vi "室外视频预览.vi"() -> ()   [LabVIEW 2018]
doc: "This example shows how to open, read, and display an AVI file in NI Vision. The VI reads the frames per second property and plays the images back at the rate specified by the AVI file."
uses:
  <vilib>/Utility/error.llb/DialogType.ctl
panel:
  out "数值输入控件":i32
  in  "重新读取":bool
  out "视频的帧数：":u32
  out "Path":path
  out "添加的路径":path
  out "视频预览":T1(plugin-control)
  in  "Stop 2":bool
  out "Progress Bar 2":i32(slide) max=41 scale=-1.0..41.0
  in  "下一步":bool
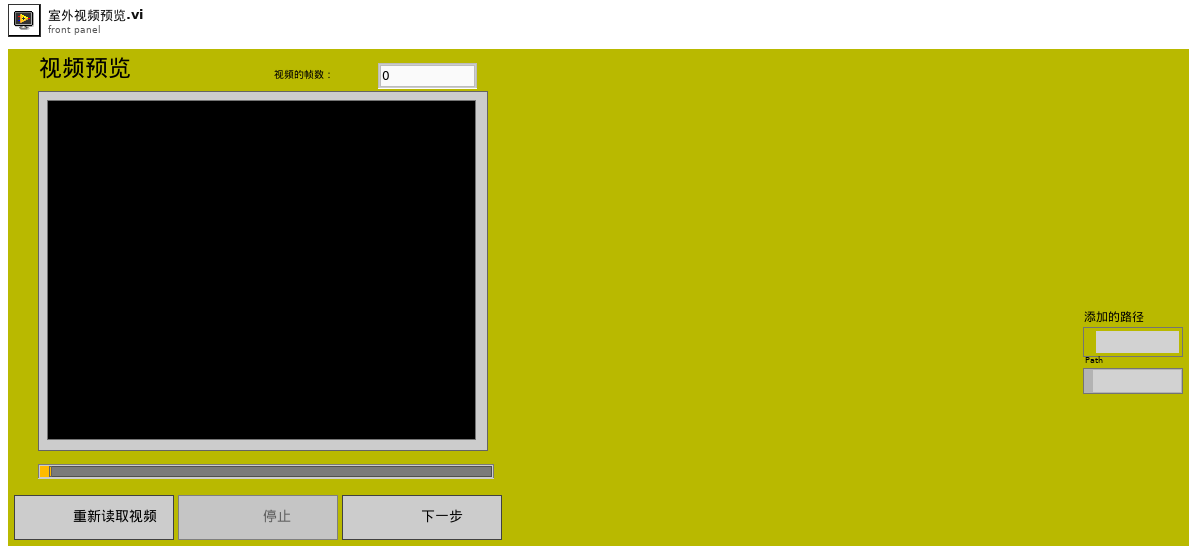
[diagram p1: front panel]
types:
  T1 = typedef "IMAQ Image.ctl" = refnum<image>
  T2 = enum8{"Enabled", "Disabled", "Disabled and Grayed Out"}
  T3 = enum32{"Invalid", "Standard", "Closed", "Hidden", "Minimized", "Maximized"}
  T4 = typedef "DialogType.ctl" = u16
  T5 = typedef "IMAQ AVI2 Refnum.ctl" = refnum<k20>
  T6 = typedef "Image Type" = u32
  T7 = cluster{"Width":u32, "Height":u32, "Frames Per Second":u32, "Codec":string, "Has Data":bool}
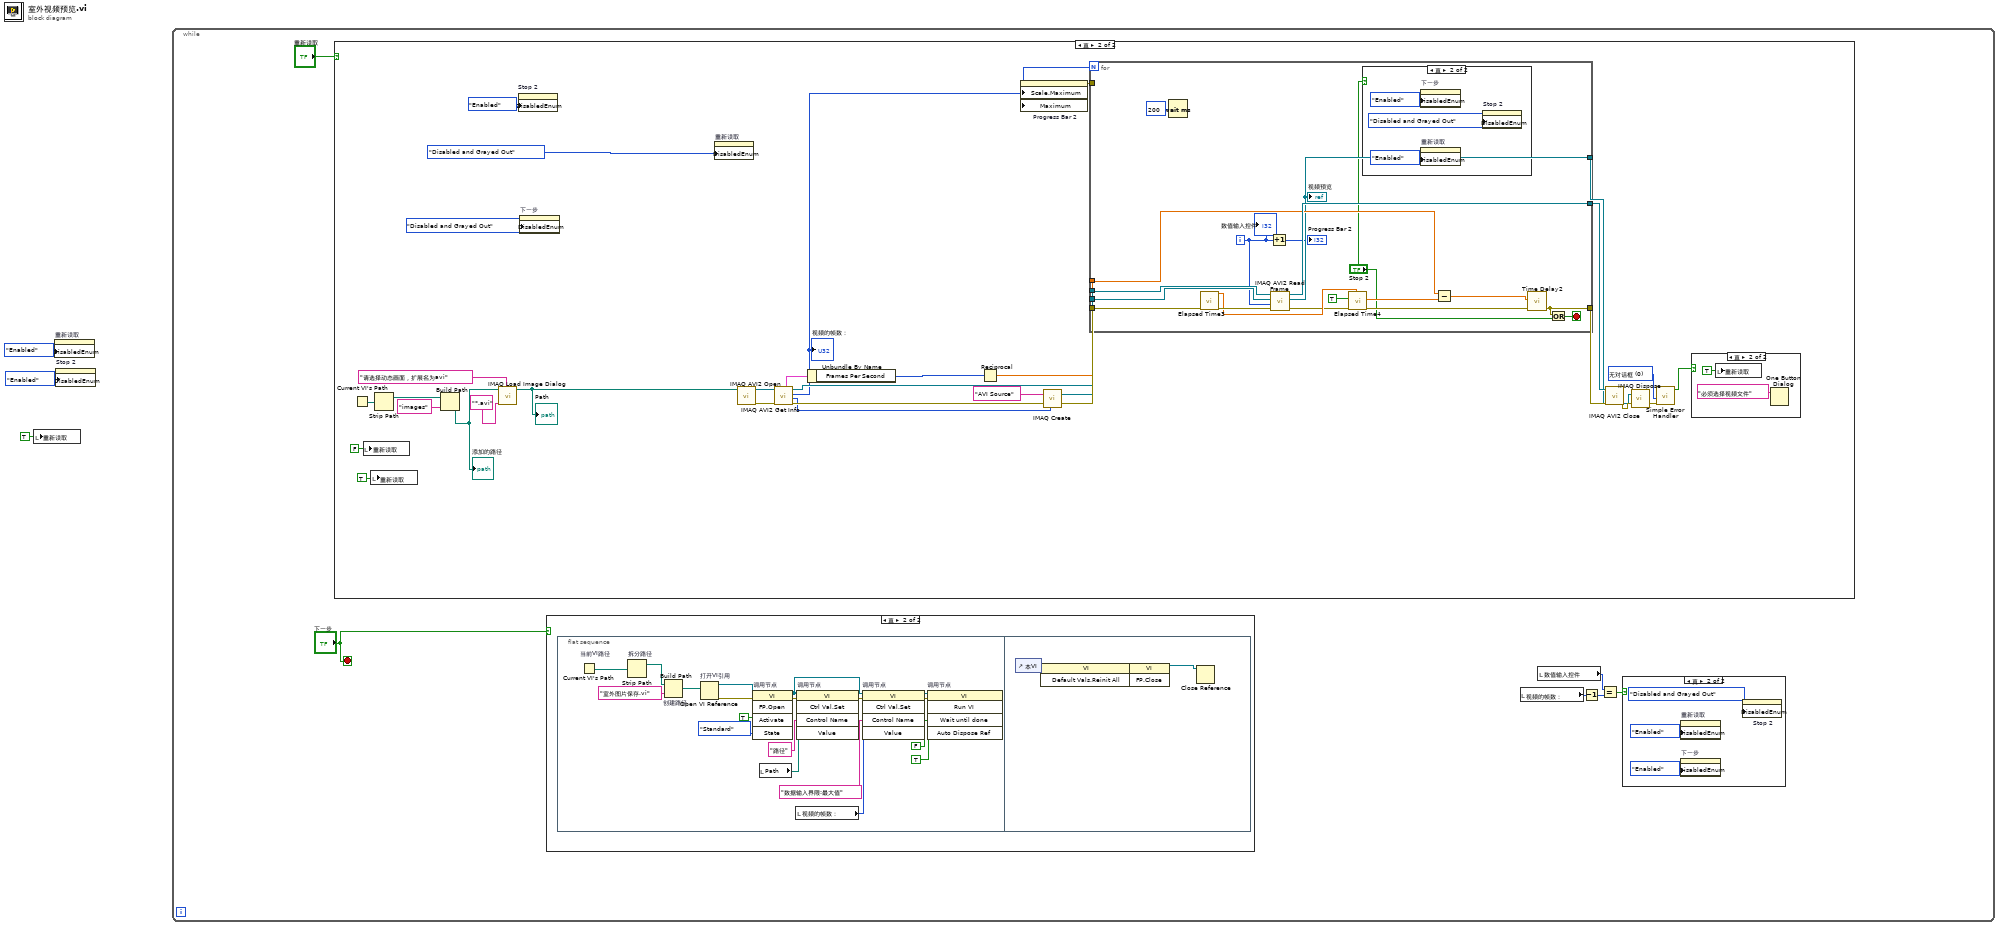
[diagram p0: block diagram]
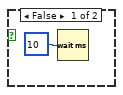
[diagram p6: hidden frame]
diagram:
  n1 = local write "重新读取"(TRUE ("布尔")) -> ()
  n2 = property on="重新读取" class="Bool (严格)"("DisabledEnum"=T2."Enabled" ("禁用")) -> ()  [unwired: 2 in, 2 out]
  n3 = property on="Stop 2" class="Bool"("DisabledEnum"=T2."Enabled" ("禁用")) -> ()  [unwired: 2 in, 2 out]
  n4 = while {
    stop <- "下一步" stop-if-true
    n5 = case shown="真" "重新读取" {
      frame False {
      }
      frame True {
        w19 = T4 0 items=["无对话框", "确定信息", "继续或停止信息", "确定信息＋警告", "继续/停止+警告"] ("type of dialog (OK msg:1)")
        n6 = Current VI's Path() -> (path=w23:path)
        n7 = local write "重新读取"(FALSE ("布尔")) -> ()
        n8 = local write "重新读取"(TRUE ("布尔")) -> ()
        n9 = Strip Path(path=w23) -> (stripped path=w22:path)  [unwired: 1 out]
        n10 = Build Path(base path=w22, name or relative path="images") -> (appended path=w26:path)
        "添加的路径" <- w26
        n11 = call "IMAQ Load Image Dialog"("Prompt"="请选择动态画面，扩展名为avi" ("prompt"), "Pattern"="*.avi", "Start Path"=w26) -> ("Path"=w20:path)  [unwired: 6 in, 2 out]
        "Path" <- w20
        n12 = property on="Stop 2" class="Bool"("DisabledEnum"=T2."Enabled" ("禁用")) -> ()  [unwired: 2 in, 2 out]
        n13 = property on="下一步" class="Bool (严格)"("DisabledEnum"=T2."Disabled and Grayed Out" ("禁用")) -> ()  [unwired: 2 in, 2 out]
        n14 = property on="重新读取" class="Bool (严格)"("DisabledEnum"=T2."Disabled and Grayed Out" ("禁用")) -> ()  [unwired: 2 in, 2 out]
        n15 = call "IMAQ AVI2 Open"("AVI File Path"=w20) -> ("error out"=w41:errorcluster, "AVI Refnum"=w40:T5)  [unwired: 2 in, 7 out]
        n16 = call "IMAQ AVI2 Get Info"("error in (no error)"=w41, "AVI Refnum"=w40) -> ("error out"=w37:errorcluster, "Image Type"=w31:T6, "Number of Frames"=w28:u32, "AVI Refnum (duplicate)"=w34:T5, "Frame Data"=w42:T7)  [unwired: 5 out]
        "视频的帧数：" <- w28
        n17 = Unbundle By Name(w42) -> ("Frames Per Second"=w30:u32)
        n18 = Reciprocal(x=w30) -> (1/x=w29:dbl)
        n19 = property on="Progress Bar 2" class="Slide (严格)"("Scale.Maximum"=w28, "Maximum"=w28) -> (error out=w27:errorcluster)  [unwired: 2 in, 1 out]
        n20 = call "IMAQ Create"("Image Name"="AVI Source", "Image Type"=w31, "error in (no error)"=w37) -> ("New Image"=w35:T1, "error out"=w36:errorcluster)  [unwired: 1 in, 1 out]
        n21 = for {
          N: w28 -> [_]
          tunnel: w35 -> [w64]
          tunnel: [w63] -> w38
          tunnel: [w52] -> w39
          tunnel: w36 -> [w62]
          tunnel: w34 -> [w65]
          tunnel: [w58] -> w32
          tunnel: w29 -> [w60]
          tunnel: w27 -> [_]
          i -> [w50]
          stop <- w51 stop-if-true
          n22 = Wait (ms)(milliseconds to wait=u32 200 ("等待时间（毫秒）")) -> ()  [unwired: 1 out]
          n23 = call "Elapsed Time3"("error in (no error)"=w62) -> ("Present (s)"=w57:dbl, "error out"=w61:errorcluster)  [unwired: 11 in, 6 out]
          n24 = Increment(x=w50) -> (x+1=→"Progress Bar 2":i32)
          n25 = call "IMAQ AVI2 Read Frame"("error in (no error)"=w61, "Frame Number"=w50, "Image"=w64, "AVI Refnum"=w65) -> ("error out"=w55:errorcluster, "Image Out"=w58:T1, "AVI Refnum (duplicate)"=w63:T5)  [unwired: 5 out]
          "视频预览" <- w58
          n26 = call "Elapsed Time4"("Reset"=TRUE, "error in (no error)"=w55, "Set Start Time (s)"=w57) -> ("Elapsed Time (s)"=w54:dbl, "error out"=w53:errorcluster)  [unwired: 9 in, 6 out]
          n27 = case shown="真" "Stop 2" {
            frame False {
            }
            frame True {
              n28 = property on="下一步" class="Bool (严格)"("DisabledEnum"=T2."Enabled" ("禁用")) -> ()  [unwired: 2 in, 2 out]
              n29 = property on="重新读取" class="Bool (严格)"("DisabledEnum"=T2."Enabled" ("禁用")) -> ()  [unwired: 2 in, 2 out]
              n30 = property on="Stop 2" class="Bool"("DisabledEnum"=T2."Disabled and Grayed Out" ("禁用")) -> ()  [unwired: 2 in, 2 out]
            }
          }
          n31 = Subtract(x=w60, y=w54) -> (x-y=w59:dbl)
          n32 = call "Time Delay2"("error in (no error)"=w53, "Delay Time (s)"=w59) -> ("error out"=w52:errorcluster)  [unwired: 9 in]
          n33 = Or(x=w52, y="Stop 2") -> (x .or. y?=w51:bool)
          "数值输入控件" <- w50
        }
        n34 = call "IMAQ AVI2 Close"("error in (no error)"=w39, "AVI Refnum"=w38) -> ("error out"=w33:errorcluster)  [unwired: 9 out]
        n35 = call "IMAQ Dispose"("Image"=w32, "error in (no error)"=w33) -> ("error out"=w43:errorcluster)  [unwired: 1 in, 3 out]
        n36 = call <vilib>:"Simple Error Handler.vi"("type of dialog (OK msg:1)"=w19, "error in (no error)"=w43) -> ("error?"=w14:bool)  [unwired: 7 out]
        n37 = case shown="真" w14 {
          frame False {
          }
          frame True {
            n38 = local write "重新读取"(TRUE ("布尔")) -> ()
            n39 = One Button Dialog(message="必须选择视频文件" ("消息")) -> ()  [unwired: 1 in, 1 out]
          }
        }
      }
    }
    n40 = case shown="真" "下一步" {
      frame False {
        n41 = Wait (ms)(milliseconds to wait=u32 10 ("等待时间（毫秒）")) -> ()  [unwired: 1 out]
      }
      frame True {
        n42 = flat-sequence {
          frame #0 {
            n43 = Current VI's Path "当前VI路径"() -> (path=w84:path)
            n44 = Strip Path "拆分路径"(path=w84) -> (stripped path=w88:path)  [unwired: 1 out]
            n45 = Build Path "创建路径"(base path=w88, name or relative path="室外图片保存.vi" ("名称或相对路径")) -> (appended path=w85:path)
            n46 = Open VI Reference "打开VI引用"(vi path=w85) -> (vi reference=w79:refnum<vi>, error out=w82:errorcluster)  [unwired: 5 in]
            n47 = invoke on="调用节点" class="VI" method="FP.Open"(reference=w79, error in=w82, "Activate"=TRUE ("激活？"), "State"=T3."Standard" ("状态")) -> (reference out=w74:refnum<vi>, error out=w70:errorcluster)  [unwired: 1 in, 3 out]
            n48 = local read "Path"() -> (w78:path)
            n49 = local read "视频的帧数："() -> (w76:u32)
            n50 = invoke on="调用节点" class="VI" method="Ctrl Val.Set"(reference=w74, error in=w70, "Control Name"="路径" ("控件名"), "Value"=w78) -> (error out=w71:errorcluster)  [unwired: 1 in, 4 out]
            n51 = invoke on="调用节点" class="VI" method="Ctrl Val.Set"(reference=w74, error in=w71, "Control Name"="数据输入界限:最大值" ("控件名"), "Value"=w76) -> (reference out=w73:refnum<vi>, error out=w72:errorcluster)  [unwired: 1 in, 3 out]
            n52 = invoke on="调用节点" class="VI" method="Run VI"(reference=w73, error in=w72, "Wait until done"=FALSE ("结束前等待"), "Auto Dispose Ref"=TRUE ("自动销毁引用")) -> ()  [unwired: 1 in, 5 out]
          }
          frame #1 {
            n53 = control-ref of="本VI"() -> (w91:refnum<vi>)
            n54 = invoke class="VI" method="Default Vals.Reinit All"(reference=w91) -> (reference out=w90:refnum<vi>)  [unwired: 2 in, 2 out]
            n55 = invoke class="VI" method="FP.Close"(reference=w90) -> (reference out=w89:refnum<vi>)  [unwired: 2 in, 2 out]
            n56 = Close Reference(reference=w89) -> ()  [unwired: 1 in, 1 out]
          }
        }
      }
    }
    n57 = local read "视频的帧数："() -> (w5:u32)
    n58 = local read "数值输入控件"() -> (w7:i32)
    n59 = Decrement(x=w5) -> (x-1=w4:u32)
    n60 = Equal?(x=w7, y=w4) -> (x = y?=w6:bool)
    n61 = case shown="真" w6 {
      frame False {
      }
      frame True {
        n62 = property on="重新读取" class="Bool (严格)"("DisabledEnum"=T2."Enabled" ("禁用")) -> ()  [unwired: 2 in, 2 out]
        n63 = property on="下一步" class="Bool (严格)"("DisabledEnum"=T2."Enabled" ("禁用")) -> ()  [unwired: 2 in, 2 out]
        n64 = property on="Stop 2" class="Bool"("DisabledEnum"=T2."Disabled and Grayed Out" ("禁用")) -> ()  [unwired: 2 in, 2 out]
      }
    }
  }
